vi "Get Version.vi"(8 "error in (no error)":errorcluster, 11 "Generic Execution Adapter in":refnum<class "Generic Execution Adapter.lvclass">) -> (0 "error out":errorcluster, 2 "Version":string, 3 "Generic Execution Adapter out":refnum<class "Generic Execution Adapter.lvclass">)   [LabVIEW 2026, in "Generic Execution Adapter.lvclass"]
uses:
  Generic Execution Adapter.lvclass
  Generic Execution Adapter.lvclass/Generic Execution Adapter.ctl
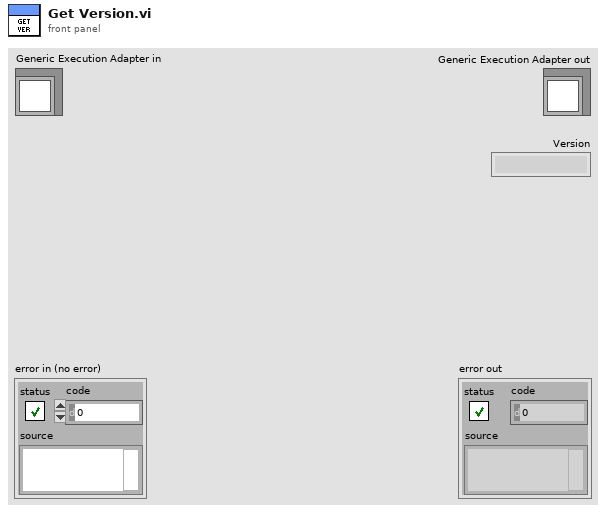
[diagram p1: front panel]
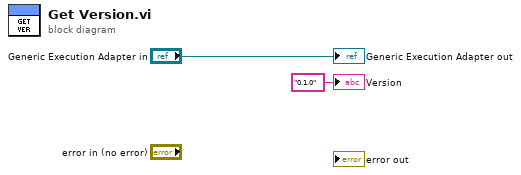
[diagram p0: block diagram]
diagram:
  "Generic Execution Adapter out" <- "Generic Execution Adapter in"
  "Version" <- "0.1.0" ("Version")
